vi "Queue Comms DeQueue.vi"(8 "error in":errorcluster) -> (0 "error out":errorcluster, 2 "element":T1)   [LabVIEW 2018, in "Display.lvlib"]
uses:
  Display.lvlib
  Private Controls/Queue FG Action.ctl
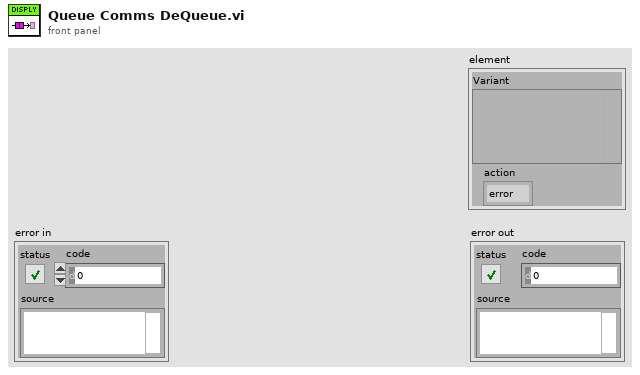
[diagram p1: front panel]
types:
  T1 = cluster{"Variant":variant, "action":enum16{"error", "exit", "init"}}
  T2 = typedef "Display.lvlib/Queue FG Action.ctl" = enum16{"Release", "Get", "Set"}
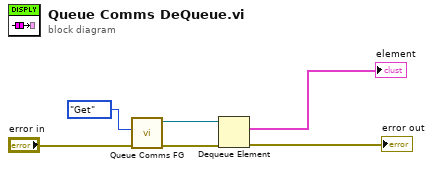
[diagram p0: block diagram]
diagram:
  n1 = call "Queue Comms FG.vi"("error in"="error in", "Action"=Queue_FG_Action."Get") -> ("error out"=w6:errorcluster, "queue out"=w5:refnum<queue>)  [unwired: 8 in]
  n2 = Dequeue Element(queue=w5, error in (no error)=w6) -> (element=→"element":T1, error out=→"error out":errorcluster)  [unwired: 1 in, 2 out]
